vi "window2.vi"(1 "Window":u16(ring) items=["Rectangular", "Bartlett-Hanning", "Blackman", "Blackman-Harris", "Blackman-Nuttall", "Bohman", "Exact Blackman", "Hamming", "Hanning", "Parzen", "Triangle", "Welch"], 2 "Unfiltered Signal":cdb[](array[numeric]), 3 "DC Offset":cdb format="%#_13g") -> (0 "Windowed Signal":cdb[](array[numeric]))   [LabVIEW 2013]
uses:
  <vilib>/Analysis/4window.llb/Hamming Window (CDB).vi
  <vilib>/Analysis/4window.llb/Hanning Window (CDB).vi
  <vilib>/Analysis/4window.llb/Welch Window (CDB).vi
  <vilib>/Analysis/4window.llb/Blackman Window (CDB).vi
  <vilib>/Analysis/4window.llb/Blackman-Harris Window (CDB).vi
  <vilib>/Analysis/4window.llb/Blackman-Nuttall Window (CDB).vi
  <vilib>/Analysis/4window.llb/Exact Blackman Window (CDB).vi
  <vilib>/Analysis/4window.llb/Modified Bartlett-Hanning Window (CDB).vi
  <vilib>/Analysis/4window.llb/Triangle Window (CDB).vi
  <vilib>/Analysis/4window.llb/Parzen Window (CDB).vi
  <vilib>/Analysis/4window.llb/Bohman Window (CDB).vi
  <vilib>/Analysis/4window.llb/AllCosWindow (CDB).vi
  <vilib>/Analysis/NI_AALPro.lvlib
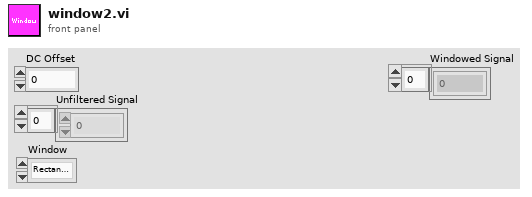
[diagram p1: front panel]
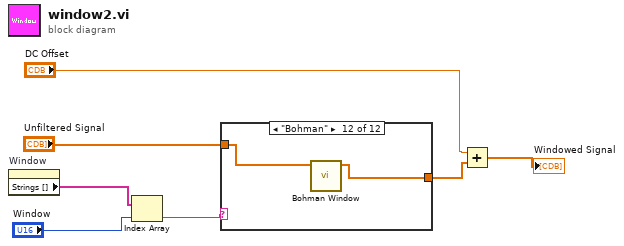
[diagram p0: block diagram]
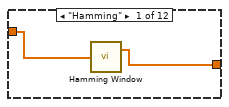
[diagram p2: hidden frame]
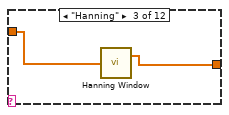
[diagram p4: hidden frame]
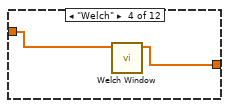
[diagram p5: hidden frame]
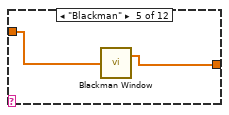
[diagram p6: hidden frame]
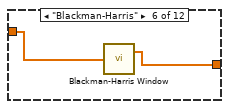
[diagram p7: hidden frame]
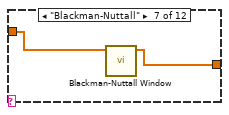
[diagram p8: hidden frame]
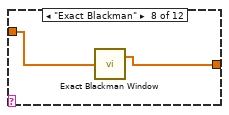
[diagram p9: hidden frame]
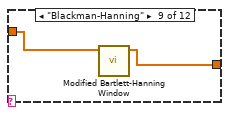
[diagram p10: hidden frame]
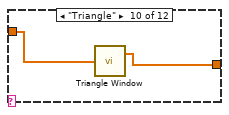
[diagram p11: hidden frame]
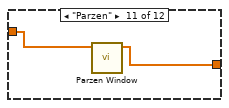
[diagram p12: hidden frame]
diagram:
  n1 = property on="Window" class="Ring (strict)"() -> ("Strings []"=w4:string[])  [unwired: 2 in, 2 out]
  n2 = Index Array(array=w4, index="Window") -> (element=w3:string)
  n3 = case shown="\"Bohman\"" w3 {
    tunnel: "Unfiltered Signal" -> [w9 w10 w12 w14 w16 w18 w20 w22 w24 w26 w28 w30]
    tunnel: [w8 w10 w11 w13 w15 w17 w19 w21 w23 w25 w27 w29] -> w1
    frame "Hamming" {
      n4 = call-poly <vilib>:"Hamming Window.vi"("X"=w9) -> ("Windowed X"=w8:cdb[])  [unwired: 1 out]
    }
    frame "False", Default {
    }
    frame "Hanning" {
      n5 = call-poly <vilib>:"Hanning Window.vi"("X"=w12) -> ("Windowed X"=w11:cdb[])  [unwired: 1 out]
    }
    frame "Welch" {
      n6 = call-poly <vilib>:"Welch Window.vi"("X"=w14) -> ("Windowed X"=w13:cdb[])  [unwired: 9 in, 1 out]
    }
    frame "Blackman" {
      n7 = call-poly <vilib>:"Blackman Window.vi"("X"=w16) -> ("Windowed X"=w15:cdb[])  [unwired: 1 out]
    }
    frame "Blackman-Harris" {
      n8 = call-poly <vilib>:"Blackman-Harris Window.vi"("X"=w18) -> ("Windowed X"=w17:cdb[])  [unwired: 1 out]
    }
    frame "Blackman-Nuttall" {
      n9 = call-poly <vilib>:"Blackman-Nuttall Window.vi"("X"=w20) -> ("Windowed X"=w19:cdb[])  [unwired: 9 in, 1 out]
    }
    frame "Exact Blackman" {
      n10 = call-poly <vilib>:"Exact Blackman Window.vi"("X"=w22) -> ("Windowed X"=w21:cdb[])  [unwired: 1 out]
    }
    frame "Blackman-Hanning" {
      n11 = call-poly <vilib>:"Modified Bartlett-Hanning Window.vi"("X"=w24) -> ("Windowed X"=w23:cdb[])  [unwired: 9 in, 1 out]
    }
    frame "Triangle" {
      n12 = call-poly <vilib>:"Triangle Window.vi"("X"=w26) -> ("Windowed X"=w25:cdb[])  [unwired: 1 out]
    }
    frame "Parzen" {
      n13 = call-poly <vilib>:"Parzen Window.vi"("X"=w28) -> ("Windowed X"=w27:cdb[])  [unwired: 9 in, 1 out]
    }
    frame "Bohman" {
      n14 = call-poly <vilib>:"Bohman Window.vi"("X"=w30) -> ("Windowed X"=w29:cdb[])  [unwired: 9 in, 1 out]
    }
  }
  n15 = Add(x="DC Offset", y=w1) -> (x+y=→"Windowed Signal":cdb[])
